vi "Messages Match.vi"(5 "Command 2":string, 7 "Command":string, 8 "error in (no error)":errorcluster, 9 "ID 1":i32, 10 "ID 2":i32, 11 "RemoteControl in":refnum<class "RemoteControl.lvclass">) -> (0 "error out":errorcluster, 3 "finished?":bool)   [LabVIEW 2019, in "RemoteControl.lvclass"]
uses:
  RemoteControl.lvclass
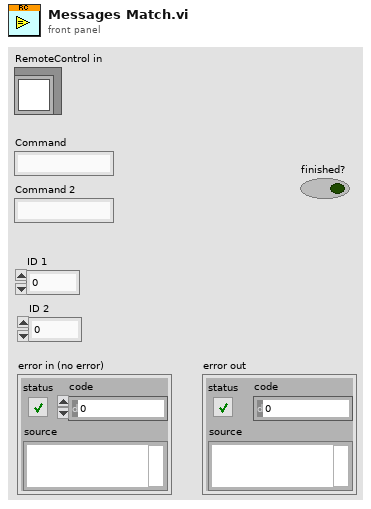
[diagram p1: front panel]
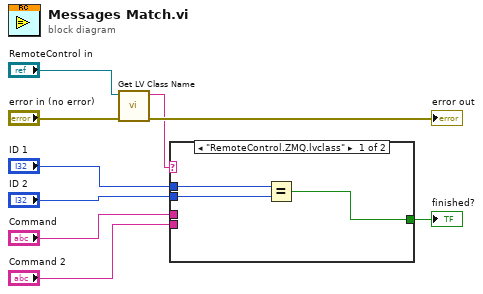
[diagram p0: block diagram]
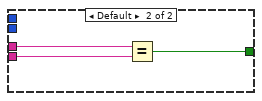
[diagram p2: hidden frame]
diagram:
  n1 = call <vilib>:"Get LV Class Name.vi"("error in (no error)"="error in (no error)", "object"="RemoteControl in") -> ("error out"=→"error out":errorcluster, "class name"=w7:string)  [unwired: 8 in]
  n2 = case shown="\"RemoteControl.ZMQ.lvclass\"" w7 {
    tunnel: "Command 2" -> [_ w15]
    tunnel: [w10 w14] -> w3
    tunnel: "Command" -> [_ w13]
    tunnel: "ID 1" -> [w12 _]
    tunnel: "ID 2" -> [w11 _]
    frame "RemoteControl.ZMQ.lvclass" {
      n3 = Equal?(x=w12, y=w11) -> (x = y?=w10:bool)
    }
    frame Default {
      n4 = Equal?(x=w13, y=w15) -> (x = y?=w14:bool)
    }
  }
  "finished?" <- w3
